vi "Gen_Sag_Swell_Anomaly.vi"(8 "Duration":i32, 9 "Amplitude":sgl, 10 "Position":dbl, 11 "Sine":sgl[](array[numeric])) -> (3 "Sine+Anomaly":sgl[](graph))   [LabVIEW 2020]
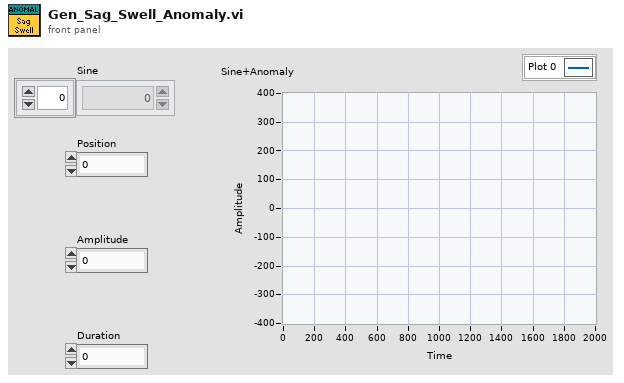
[diagram p1: front panel]
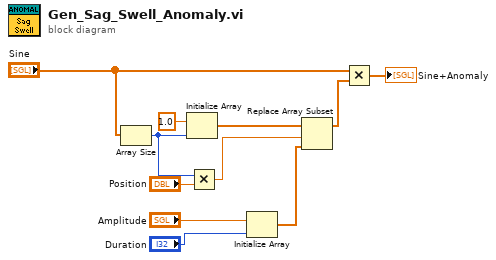
[diagram p0: block diagram]
diagram:
  n1 = Array Size(array="Sine") -> (size(s)=w5:i32)
  n2 = Initialize Array(sgl 1.0 ("element"), w5) -> (w8:sgl[])
  n3 = Multiply(x=w5, y="Position") -> (x*y=w10:dbl)
  n4 = Initialize Array("Amplitude", "Duration") -> (w7:sgl[])
  n5 = Replace Array Subset(array=w8, new element=w7, index=w10) -> (w6:sgl[])
  n6 = Multiply(x="Sine", y=w6) -> (x*y=→"Sine+Anomaly":sgl[])
